vi "DO Create.vi"(8 "error in (no error)":errorcluster, 10 "Digital Configuration Parameters":T1, 11 "Mech Pump in":refnum<class "Mech Pump.lvclass">) -> (0 "error out":errorcluster, 3 "Mech Pump out":refnum<class "Mech Pump.lvclass">)   [LabVIEW 2021, in "Mech Pump.lvclass"]
uses:
  Mech Pump.lvclass
  <vilib>/NathanCo/Digital-Tasks/Utilities/Digital Configuration Parameters.ctl
  Mech Pump.lvclass/Mech Pump.ctl
  <vilib>/NathanCo/Digital-Tasks/Digital Output/Digital Output/Digital Output.lvclass
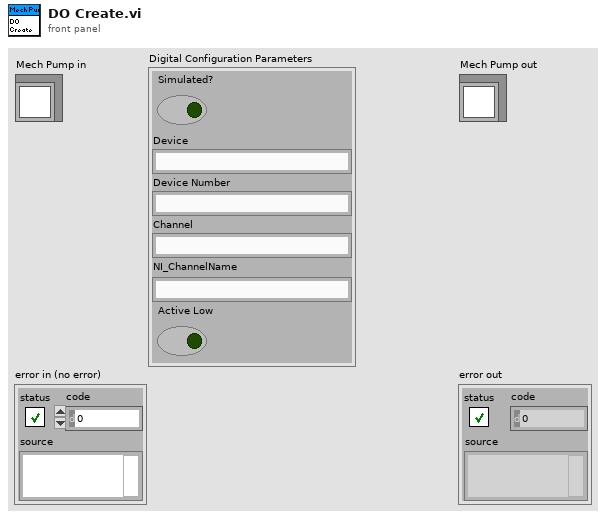
[diagram p1: front panel]
types:
  T1 = typedef "Digital Configuration Parameters.ctl" = cluster{"Simulated?":bool, "Device":string, "Device Number":string, "Channel":string, "NI_ChannelName":string, "Active Low":bool}
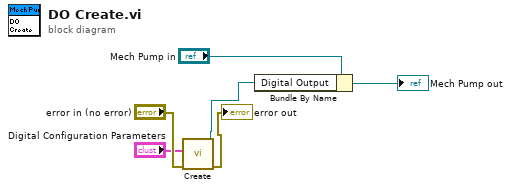
[diagram p0: block diagram]
diagram:
  n1 = call <vilib>:"Create.vi"("error in (no error)"="error in (no error)", "Digital Configuration Parameters"="Digital Configuration Parameters") -> ("error out"=→"error out":errorcluster, "Digital Output out"=w2:refnum<class "Digital Output.lvclass">)  [unwired: 8 in]
  n2 = Bundle By Name(cluster="Mech Pump in", "Digital Output"=w2) -> (→"Mech Pump out":refnum<class "Mech Pump.lvclass">)
